vi "delta Phase.vi"(10 "Phase/s [kHz]":dbl, 11 "Tranfer speed":T1) -> (3 "phase per sample (rad)":dbl=1e-06 format="%#_13g")   [LabVIEW 2018]
uses:
  controls/host_transfer_speed.ctl
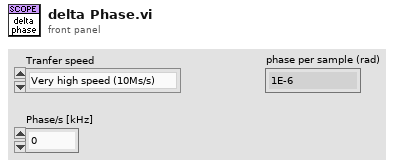
[diagram p1: front panel]
types:
  T1 = typedef "host_transfer_speed.ctl" = enum16{"Very high speed (10Ms/s)", "High speed (1Ms/s)", "Low speed (50kS/s)", "Ultra low speed (20kS/s)"}
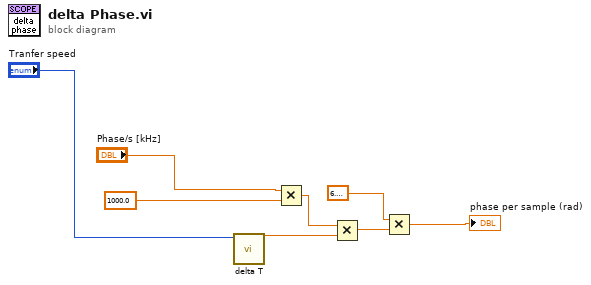
[diagram p0: block diagram]
diagram:
  n1 = call "delta T.vi"("Tranfer speed"="Tranfer speed") -> ("dt"=w2:dbl)  [unwired: 10 in]
  n2 = Multiply(x="Phase/s [kHz]", y=1000.0) -> (x*y=w3:dbl)
  n3 = Multiply(x=w3, y=w2) -> (x*y=w7:dbl)
  n4 = Multiply(x=6.283185307179586, y=w7) -> (x*y=→"phase per sample (rad)":dbl)
